vi "Controller Operation Mode Management Loop.vi"(7 "Sync Objects":T1, 8 "error in (no error)":errorcluster, 11 "FOFB Configuration":T5={"FOFB Parameters"={"Network"={"FOFB Controller IP"="", "LNLS Control Network IP"="", "LNLS Control Network Power Supplies TCP Port"=0, "LNLS Control Network FOFB Configuration TCP Port"=0, "Data Server TCP Port"=0, "Monitoring Data TCP Port"=0, "Configuration GUI TCP Port"=0, "TCP Listening Timeout"=0}, "Fast Acquisition"={"Acquisition Period"=0, "Data Buffer Size"=0}, "Response Matrix Measurement"={"Step Amplitude"=0.0, "Time Between Steps"=0, "Step Duration"=0, "Number of Averages"=0}, "Correction Algorithm"={"Correction Period"=0, "Reference Orbit Path"=path "", "Response Matrix Path"=path "", "Correction Matrix Path"=path "", "Horizontal Correction Factor"=0.0, "Vertical Correction Factor"=0.0, "Beam Current FOFB Threshold"=0.0, "Decouple H-V"=FALSE}, "Acquisition Network"=[], "Actuation Network"=[]}, "Number of Acquisition Chassis"=0, "Number of Actuation Chassis"=0, "Number of BPM Readings"=0, "BPM Reading Names"=[], "Selected BPM Readings"=[0, 1, 2, 3, 4, 5, 6, 7, 8, 9, 10, 11, 12, 13, 14, 15, 16, 17, 18, 19, 20, 21, 22, 23, 24, 25, 26, 27, 28, 29, 30, 31, 32, 33, 34, 35, 36, 37, 38, 39, 40, 41, 42, 43, 44, 45, 46, 47, 48, 49], "Number of Correctors"=0, "Corrector Names"=[], "Selected Correctors"=[0, 1, 2, 3, 4, 5, 6, 7, 8, 9, 10, 11, 12, 13, 14, 15, 16, 17, 18, 19, 20, 21, 22, 23, 24, 25, 26, 27, 28, 29, 30, 31, 32, 33, 34, 35, 36, 37, 38, 39, 40, 41, 42, 43, 44, 45, 46, 47, 48, 49], "Reference Orbit"=[], "Response Matrix"=[], "Correction Matrix"=[], "Acquisition Chassis Names"=[], "Actuation Chassis Names"=[], "Acquisition Variables"=[], "Actuation Variables"=[], "PS Matrix Mapping"=[], "Inverse PS Matrix Mapping"=[], "Response Matrix Beam Energy (MeV)"=0.0, "PID Parameters"=[], "BPM Planes"=[], "Corrector Planes"=[], "RMM Step Factor"=[]}) -> (0 "error out":errorcluster)   [LabVIEW 2011, in "Controller VIs.lvlib"]
uses:
  Controller VIs.lvlib
  Types Definitions/Type FOFB Configuration.ctl
  Types Definitions/Type FOFB Parameters.ctl
  Types Definitions/Type Network Configuration.ctl
  Types Definitions/Type FA Configuration.ctl
  Types Definitions/Type Response Matrix Measurement Configuration.ctl
  Types Definitions/Type Correction Algorithm Configuration.ctl
  Types Definitions/Type Acquisition Network Configuration.ctl
  Types Definitions/Type Actuation Network Configuration.ctl
  Types Definitions/Type PID Parameters.ctl
  Types Definitions/Type Synchronization Objects.ctl
  Types Definitions/Type Blocking Synchronization Objects.ctl
  Types Definitions/Type FA Request Parameters.ctl
  Types Definitions/Type BPM and PS select cluster.ctl
  Types Definitions/Type FA File Parameters.ctl
  Types Definitions/Type Monitoring Data.ctl
  Types Definitions/Type Diagnostics Data.ctl
  Types Definitions/Type CPU Loads Array.ctl
  Types Definitions/Type CPU Loads.ctl
  Types Definitions/Type Non-blocking Synchronization Objects.ctl
  Types Definitions/Type FOFB Variables.ctl
  Types Definitions/Type Actuation State.ctl
  <vilib>/Platform/TimedLoop/XDataNode/timing_clust.ctl
  <vilib>/Platform/TimedLoop/XDataNode/nitl_modes.ctl
  <vilib>/Platform/TimedLoop/XDataNode/wakeup.ctl
  Controller Global Variables/LNLS Control FOFB Configuration In.vi
  Controller Global Variables/Controller Operation Mode.vi
  Controller Global Variables/LNLS Control FOFB Configuration Out.vi
  <vilib>/Platform/TimedLoop/XDataNode/XDataNode.xnode
  Type Definitions.lvlib
  Controller Global Variables.lvlib
  <vilib>/Platform/TimedLoop/XDataNode/XDNodeRunTimeDep.lvlib
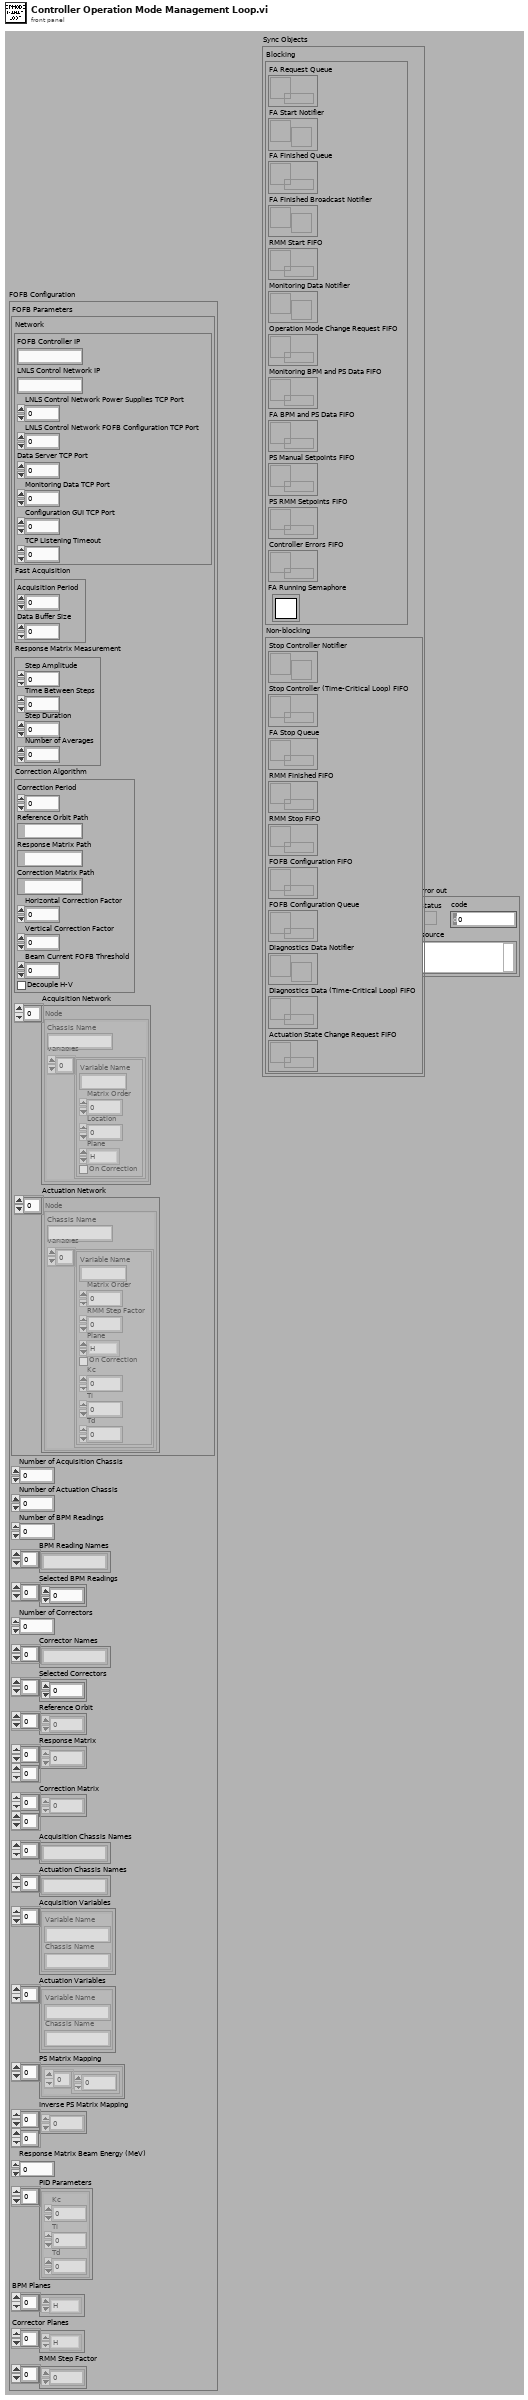
[diagram p1: front panel]
types:
  T1 = typedef "Type Definitions.lvlib/Type Synchronization Objects.ctl" = cluster{"Blocking":T2, "Non-blocking":T4}
  T2 = typedef "Type Definitions.lvlib/Type Blocking Synchronization Objects.ctl" = cluster{"FA Request Queue":refnum<queue>, "FA Start Notifier":refnum<notifier>, "FA Finished Queue":refnum<queue>, "FA Finished Broadcast Notifier":refnum<notifier>, "RMM Start FIFO":refnum<k33>, "Monitoring Data Notifier":refnum<notifier>, "Operation Mode Change Request FIFO":refnum<k33>, "Monitoring BPM and PS Data FIFO":refnum<k33>, "FA BPM and PS Data FIFO":refnum<k33>, "PS Manual Setpoints FIFO":refnum<k33>, "PS RMM Setpoints FIFO":refnum<k33>, "Controller Errors FIFO":refnum<k33>, "FA Running Semaphore":T3}
  T3 = typedef "Semaphore RefNum" = refnum<k1>
  T4 = typedef "Type Definitions.lvlib/Type Non-blocking Synchronization Objects.ctl" = cluster{"Stop Controller Notifier":refnum<notifier>, "Stop Controller (Time-Critical Loop) FIFO":refnum<k33>, "FA Stop Queue":refnum<queue>, "RMM Finished FIFO":refnum<k33>, "RMM Stop FIFO":refnum<k33>, "FOFB Configuration FIFO":refnum<k33>, "FOFB Configuration Queue":refnum<queue>, "Diagnostics Data Notifier":refnum<notifier>, "Diagnostics Data (Time-Critical Loop) FIFO":refnum<k33>, "Actuation State Change Request FIFO":refnum<k33>}
  T5 = typedef "Type Definitions.lvlib/Type FOFB Configuration.ctl" = cluster{"FOFB Parameters":T6, "Number of Acquisition Chassis":i32, "Number of Actuation Chassis":i32, "Number of BPM Readings":i32, "BPM Reading Names":string[], "Selected BPM Readings":u32[], "Number of Correctors":i32, "Corrector Names":string[], "Selected Correctors":u32[], "Reference Orbit":dbl[], "Response Matrix":dbl[][], "Correction Matrix":dbl[][], "Acquisition Chassis Names":string[], "Actuation Chassis Names":string[], "Acquisition Variables":cluster{"Variable Name":string, "Chassis Name":string}[], "Actuation Variables":cluster{"Variable Name":string, "Chassis Name":string}[], "PS Matrix Mapping":cluster{u32[]}[], "Inverse PS Matrix Mapping":u32[][], "Response Matrix Beam Energy (MeV)":dbl, "PID Parameters":T13[], "BPM Planes":enum8{"H", "V"}[], "Corrector Planes":enum8{"H", "V"}[], "RMM Step Factor":dbl[]}
  T6 = typedef "Type Definitions.lvlib/Type FOFB Parameters.ctl" = cluster{"Network":T7, "Fast Acquisition":T8, "Response Matrix Measurement":T9, "Correction Algorithm":T10, "Acquisition Network":T11, "Actuation Network":T12}
  T7 = typedef "Type Definitions.lvlib/Type Network Configuration.ctl" = cluster{"FOFB Controller IP":string, "LNLS Control Network IP":string, "LNLS Control Network Power Supplies TCP Port":u16, "LNLS Control Network FOFB Configuration TCP Port":u16, "Data Server TCP Port":u16, "Monitoring Data TCP Port":u16, "Configuration GUI TCP Port":u16, "TCP Listening Timeout":i32}
  T8 = typedef "Type Definitions.lvlib/Type FA Configuration.ctl" = cluster{"Acquisition Period":u32, "Data Buffer Size":u32}
  T9 = typedef "Type Definitions.lvlib/Type Response Matrix Measurement Configuration.ctl" = cluster{"Step Amplitude":dbl, "Time Between Steps":u32, "Step Duration":u32, "Number of Averages":u32}
  T10 = typedef "Type Definitions.lvlib/Type Correction Algorithm Configuration.ctl" = cluster{"Correction Period":u32, "Reference Orbit Path":path, "Response Matrix Path":path, "Correction Matrix Path":path, "Horizontal Correction Factor":dbl, "Vertical Correction Factor":dbl, "Beam Current FOFB Threshold":dbl, "Decouple H-V":bool}
  T11 = typedef "Type Definitions.lvlib/Type Acquisition Network Configuration.ctl" = cluster{"Chassis Name":string, "Variables":cluster{"Variable Name":string, "Matrix Order":u32, "Location":dbl, "Plane":enum8{"H", "V"}, "On Correction":bool}[]}[]
  T12 = typedef "Type Definitions.lvlib/Type Actuation Network Configuration.ctl" = cluster{"Chassis Name":string, "Variables":cluster{"Variable Name":string, "Matrix Order":u32, "RMM Step Factor":dbl, "Plane":enum8{"H", "V"}, "On Correction":bool, "Kc":dbl, "Ti":dbl, "Td":dbl}[]}[]
  T13 = typedef "Type Definitions.lvlib/Type PID Parameters.ctl" = cluster{"Kc":fxp<+/-,16,8>, "Ti":fxp<+/-,16,8>, "Td":fxp<+/-,16,8>}
  T14 = enum16{"Idle Mode", "Error Mode", "Manual Mode", "FOFB Mode", "RMM Mode"}
  T15 = typedef "XDNodeRunTimeDep.lvlib/timing_clust.ctl" = cluster{"Expected End [f-1]":u64, "Actual End [f-1]":u64, "Finished Late? [f-1]":bool, "Expected End [i-1]":u64, "Actual End [i-1]":u64, "Finished Late? [i-1]":bool, "Expected Start [i]":u64, "Actual Start [i]":u64, "Expected Start [f]":u64, "Actual Start [f]":u64, "Source Name":string, "Structure Name":string, "Period":i64, "Deadline":i64, "Offset":i64, "Start":i64, "Priority":i32, "Timeout":i32, "Mode":T16, "Wakeup Reason":T17, "Error":errorcluster, "Source Type":string, "Secondary Source Type":string, "Global End Time":u64, "Global Start Time":u64, "Frame Duration":u64, "Iteration Duration":u64, "Assigned CPU":i32, "I/O Scan Engine Mode":u32}
  T16 = typedef "XDNodeRunTimeDep.lvlib/nitl_modes.ctl" = enum32{"No Change", "Process missed periods, maintain original phase", "Discard missed periods, maintain original phase", "Process missed periods, ignore original phase", "Discard missed periods, ignore original phase"}
  T17 = typedef "XDNodeRunTimeDep.lvlib/wakeup.ctl" = enum32{"Normal", "Aborted", "Asynchronous wakeup", "Timing source error", "Timed loop error", "Timeout"}
  T18 = typedef "Type Definitions.lvlib/Type Actuation State.ctl" = enum16{"Only reading", "Manual", "FOFB Initialization", "FOFB", "FOFB Stopping", "RMM Initialization", "RMM", "RMM Stopping"}
  T19 = cluster{"Operation Mode":enum16{"Idle Mode", "Error Mode", "Manual Mode", "FOFB Mode", "RMM Mode"}, "Correction Period (usec)":i32, "Beam Energy (MeV)":sgl, "Beam Current (mA)":sgl}
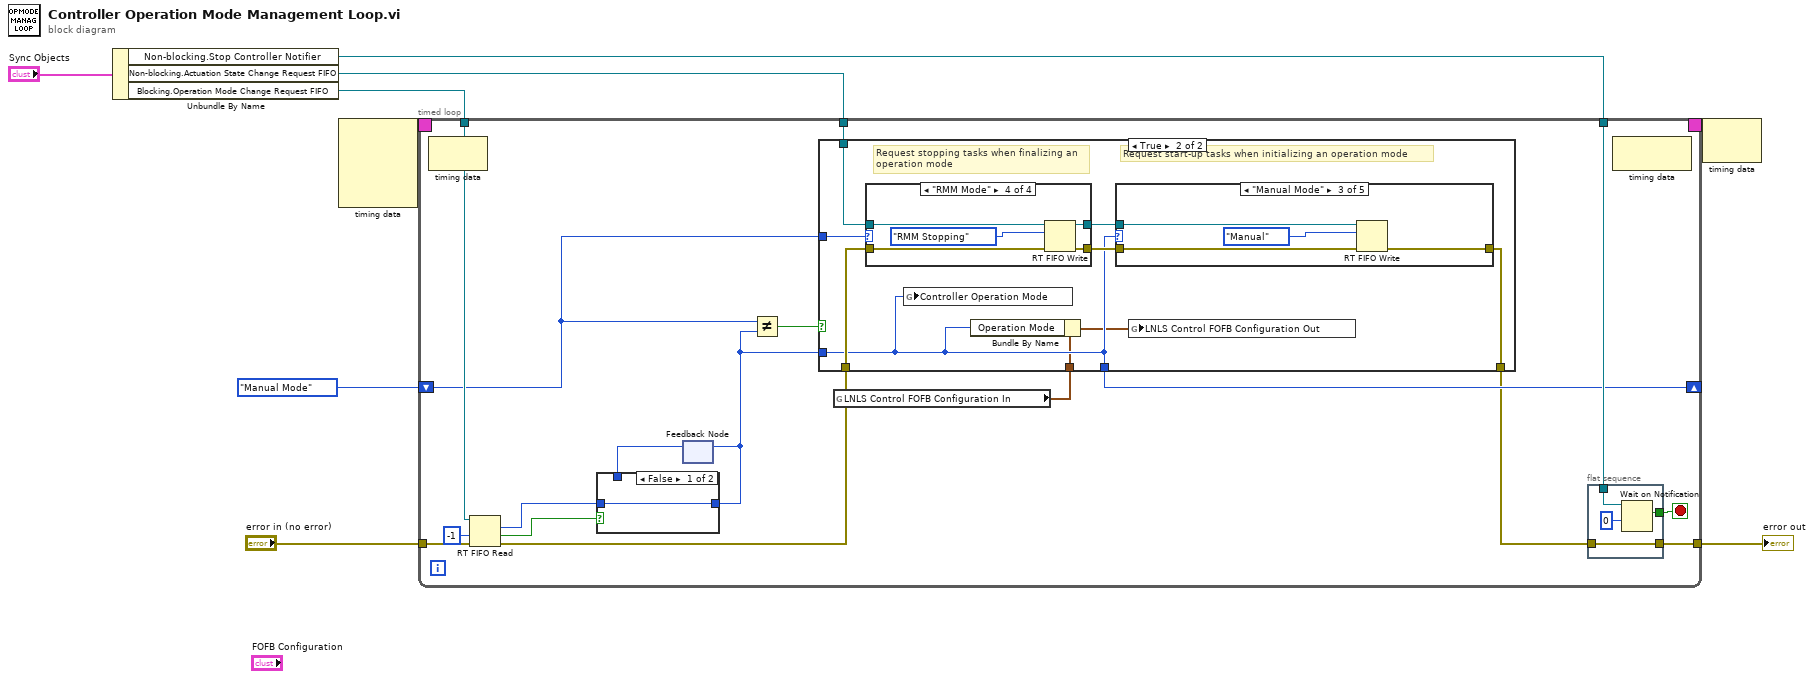
[diagram p0: block diagram]
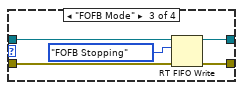
[diagram p5: hidden frame]
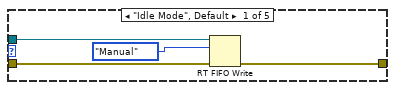
[diagram p6: hidden frame]
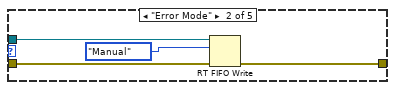
[diagram p7: hidden frame]
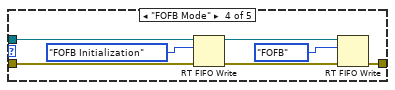
[diagram p8: hidden frame]
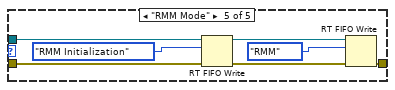
[diagram p9: hidden frame]
diagram:
  n1 = Unbundle By Name("Sync Objects") -> ("Non-blocking.Stop Controller Notifier"=w7:refnum<notifier>, "Non-blocking.Actuation State Change Request FIFO"=w3:refnum<k33>, "Blocking.Operation Mode Change Request FIFO"=w6:refnum<k33>)
  n2 = node-c288() -> (w2:T15)  [unwired: 4 in]
  n3 = timed-loop {
    tunnel: [w19] -> w9
    tunnel: "error in (no error)" -> [w22]
    tunnel: w7 -> [w25]
    shift-right: [w21] -> _
    shift-left: T14."Manual Mode" ("Operation Mode") -> [w17]
    tunnel: w6 -> [w24]
    tunnel: w3 -> [w20]
    timing: w2 -> [_]
    timing-out: [_] -> w1
    stop <- w26 stop-if-true
    n4 = node-c288() -> ()  [unwired: 1 in, 1 out]
    n5 = RT FIFO Read(0:w24, 2:-1 ("timeout in ms (0)"), 3:w22) -> (9:w15:T14, 10:w14:bool, 11:w23:errorcluster)  [unwired: 1 in, 2 out]
    n6 = feedback #1() -> (w16:T14)  [unwired: 1 in]
    n7 = case shown="False" w14 {
      tunnel: [w80 w81] -> w12
      tunnel: w15 -> [w80 _]
      tunnel: w16 -> [_ w81]
      frame False {
      }
      frame True {
      }
    }
    n8 = feedback-in #1(w12) -> ()
    n9 = Not Equal?(x=w17, y=w12) -> (x != y?=w13:bool)
    n10 = global read "LNLS Control FOFB Configuration In.vi" "LNLS Control FOFB Configuration In"() -> (w10:T19)
    n11 = case shown="True" w13 {
      tunnel: [w30 w33] -> w21
      tunnel: w17 -> [w30 w38]
      tunnel: w12 -> [_ w33]
      tunnel: [w29 w35] -> w18
      tunnel: w20 -> [_ w39]
      tunnel: w23 -> [w29 w34]
      tunnel: w10 -> [_ w32]
      frame False {
      }
      frame True {
        # "Request start-up tasks when initializing an operation mode"
        # "Request stopping tasks when finalizing an operation mode"
        n12 = case shown="\"RMM Mode\"" w38 {
          tunnel: w39 -> [w40 w42 w48 w53]
          tunnel: w34 -> [w41 w43 w47 w52]
          tunnel: [w41 w43 w46 w51] -> w36
          tunnel: [w40 w42 w45 w50] -> w37
          frame "Idle Mode", Default {
          }
          frame "Manual Mode" {
          }
          frame "FOFB Mode" {
            n13 = RT FIFO Write(0:w48, 1:Type_Actuation_State."FOFB Stopping" ("element"), 3:w47) -> (8:w45:refnum<k33>, 11:w46:errorcluster)  [unwired: 2 in, 2 out]
          }
          frame "RMM Mode" {
            n14 = RT FIFO Write(0:w53, 1:Type_Actuation_State."RMM Stopping" ("element"), 3:w52) -> (8:w50:refnum<k33>, 11:w51:errorcluster)  [unwired: 2 in, 2 out]
          }
        }
        n15 = global write "Controller Operation Mode.vi" "Controller Operation Mode"(w33) -> ()
        n16 = Bundle By Name(cluster=w32, "Operation Mode"=w33) -> (w31:T19)
        n17 = case shown="\"Manual Mode\"" w33 {
          tunnel: w37 -> [w57 w60 w64 w70 w79]
          tunnel: w36 -> [w56 w61 w65 w69 w77]
          tunnel: [w55 w59 w63 w68 w75] -> w35
          frame "Idle Mode", Default {
            n18 = RT FIFO Write(0:w57, 1:Type_Actuation_State."Manual" ("element"), 3:w56) -> (11:w55:errorcluster)  [unwired: 2 in, 3 out]
          }
          frame "Error Mode" {
            n19 = RT FIFO Write(0:w60, 1:Type_Actuation_State."Manual" ("element"), 3:w61) -> (11:w59:errorcluster)  [unwired: 2 in, 3 out]
          }
          frame "Manual Mode" {
            n20 = RT FIFO Write(0:w64, 1:Type_Actuation_State."Manual" ("element"), 3:w65) -> (11:w63:errorcluster)  [unwired: 2 in, 3 out]
          }
          frame "FOFB Mode" {
            n21 = RT FIFO Write(0:w70, 1:Type_Actuation_State."FOFB Initialization" ("element"), 3:w69) -> (8:w72:refnum<k33>, 11:w71:errorcluster)  [unwired: 2 in, 2 out]
            n22 = RT FIFO Write(0:w72, 1:Type_Actuation_State."FOFB" ("element"), 3:w71) -> (11:w68:errorcluster)  [unwired: 2 in, 3 out]
          }
          frame "RMM Mode" {
            n23 = RT FIFO Write(0:w79, 1:Type_Actuation_State."RMM Initialization" ("element"), 3:w77) -> (8:w78:refnum<k33>, 11:w76:errorcluster)  [unwired: 2 in, 2 out]
            n24 = RT FIFO Write(0:w78, 1:Type_Actuation_State."RMM" ("element"), 3:w76) -> (11:w75:errorcluster)  [unwired: 2 in, 3 out]
          }
        }
        n25 = global write "LNLS Control FOFB Configuration Out.vi" "LNLS Control FOFB Configuration Out"(w31) -> ()
      }
    }
    n26 = flat-sequence {
      tunnel: [w85] -> w26
      tunnel: w25 -> [w84]
      tunnel: [w82] -> w19
      tunnel: w18 -> [w82]
      frame #0 {
        n27 = Wait on Notification(notifier=w84, timeout in ms (-1)=0) -> (notification=w85:bool)  [unwired: 2 in, 3 out]
      }
    }
    n28 = node-c288() -> ()  [unwired: 1 in, 1 out]
  }
  "error out" <- w9
  n29 = node-c288(w1) -> ()  [unwired: 1 out]
